vi "Import DPIDs.vi"(8 "error in (no error)":errorcluster, 11 "Node Ptr":u64 format="%.0x") -> (0 "error out":errorcluster)   [LabVIEW 2024, in "Diagnostics Addon System Explorer.lvlib"]
uses:
  Diagnostics Addon System Explorer.lvlib
  Addon Shared/Types/DPID.ctl
  Addon Shared/Types/DPID.Rate.ctl
  Addon Shared/Types/Type.ctl
  <vilib>/Utility/error.llb/Trim Whitespace One-Sided.vi
  <vilib>/NI VeriStand/Custom Device API/Custom Device API.lvlib
  <vilib>/NI VeriStand/Custom Device Tools/Custom Device Utility Library/Custom Device Utility Library.lvlib
  Addon Shared/Diagnostics Addon Shared.lvlib
panel:
  in  "Tag":string
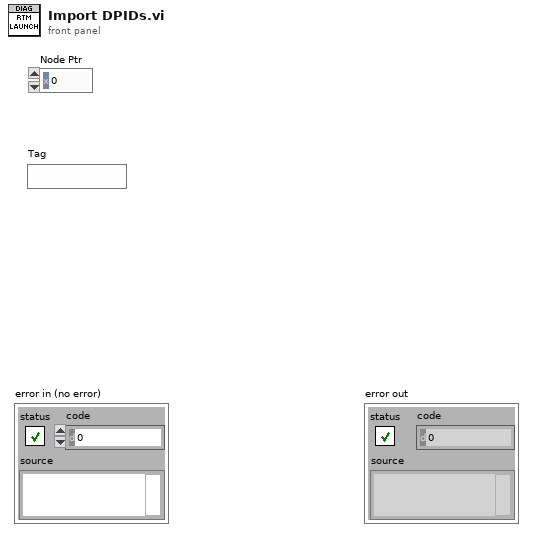
[diagram p1: front panel]
types:
  T1 = typedef "Diagnostics Addon Shared.lvlib/DPID.ctl" = cluster{"DPID ID":u8, "Speed":T2, "PIDs":u16[]}
  T2 = typedef "Diagnostics Addon Shared.lvlib/DPID.Rate.ctl" = enum16{"Slow", "Medium", "Fast"}
  T3 = typedef "Diagnostics Addon Shared.lvlib/Type.ctl" = enum16{"DID", "CDID", "PID", "CPID", "Read Memory", "Write Memory", "IO Control", "Routine Start", "Routine Request", "Routine Stop", "User Defined", "DTC Control", "Clear DTCs", "Read DTCs", "Start DTCs", "DTC Change Count", "Tester Present", "Unlock ECU", "Reset ECU", "Diag Session Control", "Communication Control", "DPID Control", "Poll Control", "Diag Comm Port Control"}
  T4 = typedef "Diagnostics Addon System Explorer.lvlib/Frame.Export.ctl" = cluster{"Name":string, "ID":u32, "Signals":T5[]}
  T5 = typedef "Diagnostics Addon Shared.lvlib/Signal.ctl" = cluster{"Start Bit":u32, "Length":u32, "Scaling Factor":dbl, "Scaling Offset":dbl, "Minimum":dbl, "Maximum":dbl, "Data Type":u32, "Byte Order":u32, "Default Value":dbl, "Name":string, "Units":string}
  T6 = typedef "Custom Device API.lvlib/Custom Device Item Ref.ctl" = u64
  T7 = typedef "Custom Device API.lvlib/Custom Device Item Info.ctl" = cluster{"Name":string, "Is Channel":bool, "GUID":string, "Is Waveform":bool}
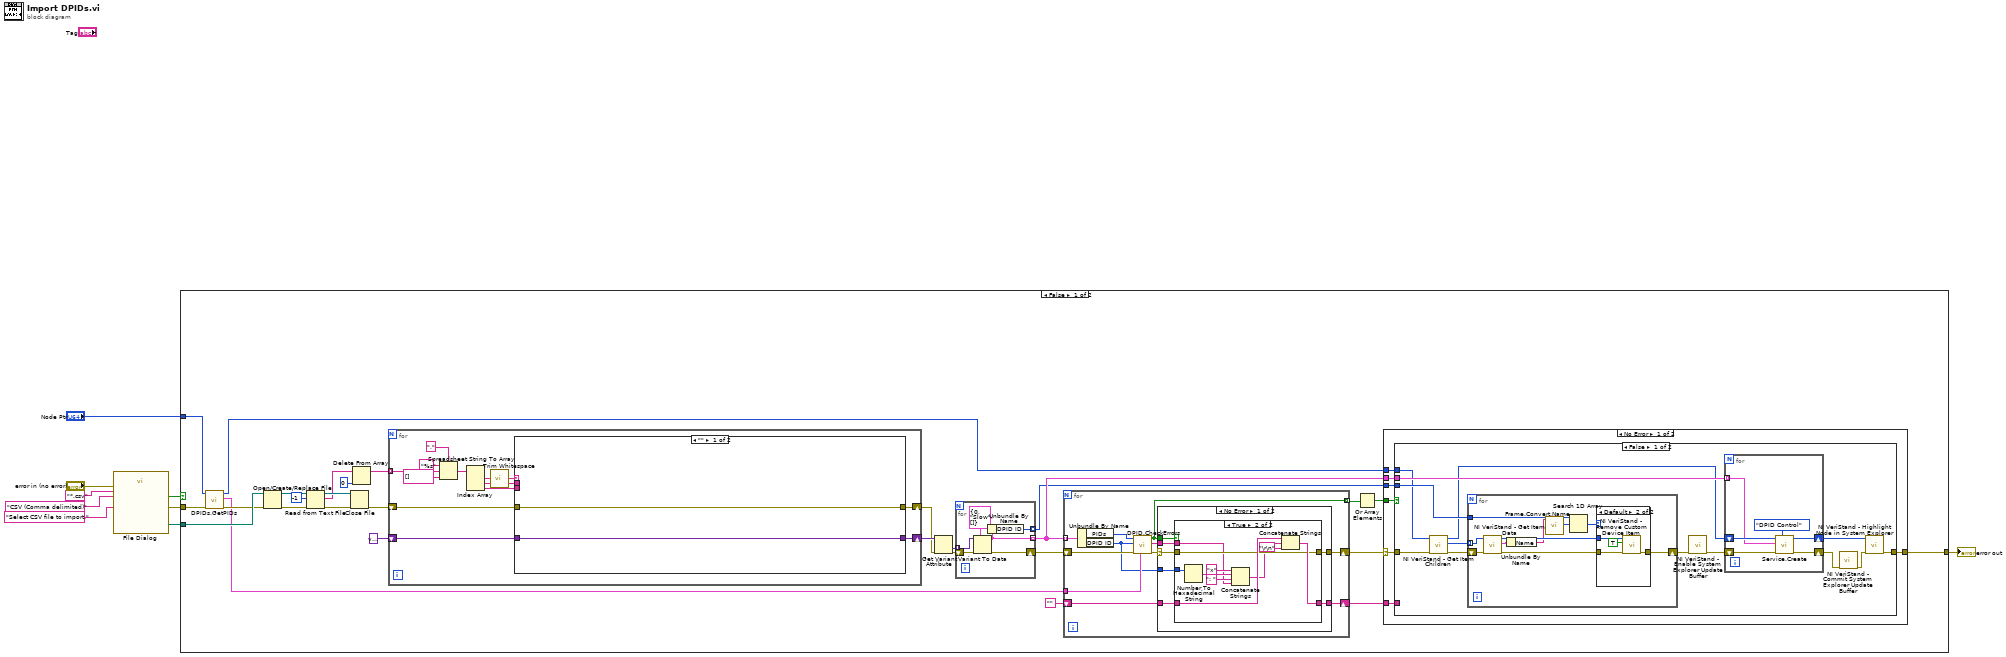
[diagram p0: block diagram]
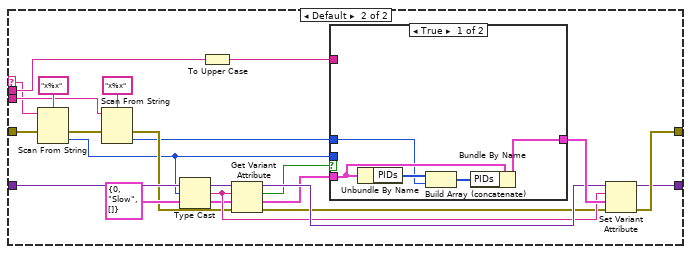
[diagram p2: hidden frame]
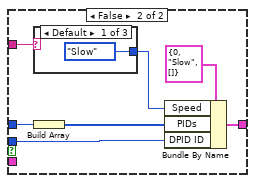
[diagram p3: hidden frame]
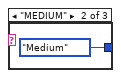
[diagram p4: hidden frame]
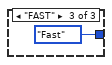
[diagram p5: hidden frame]
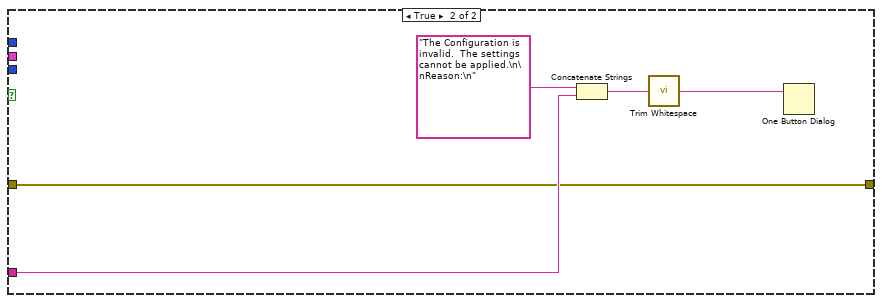
[diagram p7: hidden frame]
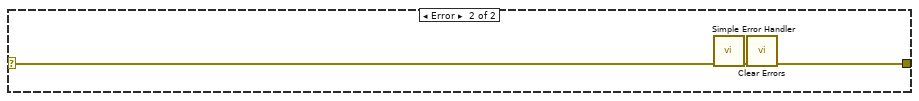
[diagram p8: hidden frame]
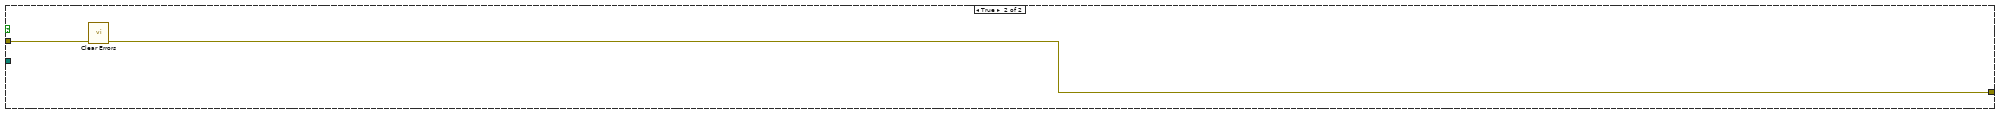
[diagram p11: hidden frame]
diagram:
  n1 = call "File Dialog"("prompt"="Select CSV file to import.", "error in"="error in (no error)", "pattern (all files)"="*.csv" ("pattern label"), "pattern label"="CSV (Comma delimited)") -> ("selected path"=w4:path, "cancelled"=w6:bool, "error out"=w5:errorcluster)  [unwired: 8 in, 1 out]
  n2 = case shown="False" w6 {
    tunnel: w5 -> [w14 w178]
    tunnel: w4 -> [w34 _]
    tunnel: "Node Ptr" -> [w12 _]
    tunnel: [w18 w177] -> w2
    frame False {
      n3 = call "DPIDs.GetPIDs.vi"("error in (no error)"=w14, "Item Ref in"=w12) -> ("error out"=w13:errorcluster, "PIDs"=w10:T4[], "Section Ref out"=w11:T6)  [unwired: 7 in]
      n4 = Open/Create/Replace File(file path (use dialog)=w34, error in=w13) -> (refnum out=w37:refnum<file>, error out=w38:errorcluster)  [unwired: 4 in, 1 out]
      n5 = Read from Text File(file (use dialog)=w37, count=-1, error in=w38) -> (refnum out=w36:refnum<file>, text=w26:string[], error out=w35:errorcluster)  [unwired: 1 in, 1 out]
      n6 = Close File(refnum=w36, error in=w35) -> (error out=w32:errorcluster)  [unwired: 1 out]
      n7 = Delete From Array(array=w26, index=0) -> (array with subset deleted=w25:string[])  [unwired: 1 in, 1 out]
      n8 = for {
        tunnel: w25 -> [w47] mode=indexing
        shift-right: [w49] -> w29
        shift-left: w32 -> [w50]
        shift-right: [w48] -> w30
        shift-left: variant -> [w51]
        n9 = Spreadsheet String To Array(delimiter (Tab)=",", format string="%s", spreadsheet string=w47, array type (2D Dbl)=string[] []) -> (array=w43:string[])
        n10 = Index Array(array=w43) -> (element #1=w40:string, element #2=w41:string, element #3=w42:string)  [unwired: 3 in]
        n11 = call <vilib>:"Trim Whitespace.vi"("string"=w40) -> ("trimmed string"=w39:string)  [unwired: 1 in]
        n12 = case shown="\"\"" w39 {
          selector: w39 -> [_ w54]
          tunnel: w51 -> [w53 w73]
          tunnel: w50 -> [w52 w72]
          tunnel: [w52 w69] -> w49
          tunnel: [w53 w68] -> w48
          tunnel: w42 -> [_ w58]
          tunnel: w41 -> [_ w57]
          frame "" {
          }
          frame Default {
            n13 = Scan From String(format string="x%x", input string=w54, error in=w72) -> (error out=w60:errorcluster, output 1=w55:u32)  [unwired: 2 in, 2 out]
            n14 = Scan From String(format string="x%x", input string=w58, error in=w60) -> (error out=w59:errorcluster, output 1=w56:u32)  [unwired: 2 in, 2 out]
            n15 = Type Cast(x=w55) -> (*(type *) &x=w67:string)  [unwired: 1 in]
            n16 = To Upper Case(1:w57) -> (0:w62:string)
            n17 = Get Variant Attribute(Variant=w73, name=w67, default value (empty Variant)=T1 {"DPID ID"=0, "Speed"=enum."Slow", "PIDs"=[]} ("DPID"), error in=w59) -> (duplicate Variant=w70:variant, found=w66:bool, value=w65:T1, error out=w63:errorcluster)
            n18 = case shown="True" w66 {
              tunnel: w55 -> [_ w80]
              tunnel: w62 -> [_ w82]
              tunnel: [w76 w86] -> w71
              tunnel: w65 -> [w79 _]
              tunnel: w56 -> [w75 w84]
              frame True {
                n19 = Unbundle By Name(w79) -> ("PIDs"=w78:u16[])
                n20 = Build Array (concatenate)(w78, w75) -> (w77:u32[])
                n21 = Bundle By Name(cluster=w79, "PIDs"=w77) -> (w76:T1)
              }
              frame False {
                n22 = case shown="Default" w82 {
                  tunnel: [DPID.Rate."Slow" ("Speed") DPID.Rate."Medium" ("Speed") DPID.Rate."Fast" ("Speed")] -> w81
                  frame Default {
                  }
                  frame "MEDIUM" {
                  }
                  frame "FAST" {
                  }
                }
                n23 = Build Array(w84) -> (w83:u32[])
                n24 = Bundle By Name(cluster=T1 {"DPID ID"=0, "Speed"=enum."Slow", "PIDs"=[]} ("DPID"), "Speed"=w81, "PIDs"=w83, "DPID ID"=w80) -> (w86:T1)
              }
            }
            n25 = Set Variant Attribute(Variant=w70, name=w67, value=w71, error in=w63) -> (Variant out=w68:variant, error out=w69:errorcluster)  [unwired: 1 out]
          }
        }
      }
      n26 = Get Variant Attribute(Variant=w30, error in=w29) -> (values=w28:variant[], error out=w27:errorcluster)  [unwired: 2 in, 2 out]
      n27 = for {
        tunnel: w28 -> [w95] mode=indexing
        shift-right: [w93] -> w17
        shift-left: w27 -> [w94]
        tunnel: [w92] -> w19 mode=indexing
        tunnel: [w91] -> w16 mode=indexing
        n28 = Variant To Data(error in=w94, type=T1 {"DPID ID"=0, "Speed"=enum."Slow", "PIDs"=[]} ("DPID"), Variant=w95) -> (data=w92:T1, error out=w93:errorcluster)
        n29 = Unbundle By Name(w92) -> ("DPID ID"=w91:u8)
      }
      n30 = for {
        tunnel: w19 -> [w155] mode=indexing
        shift-right: [w152] -> w15
        shift-left: w17 -> [w151]
        shift-right: [w154] -> w20
        shift-left: "" -> [w153]
        tunnel: [w148] -> w22 mode=indexing
        tunnel: w10 -> [w147]
        n31 = Unbundle By Name(w155) -> ("PIDs"=w146:u16[], "DPID ID"=w145:u8)
        n32 = call "DPID.CheckErrors.vi"("Existing PIDs"=w147, "error in (no error)"=w151, "DPID ID"=w145, "PIDs"=w146) -> ("error out"=w150:errorcluster, "Reason"=w149:string, "Error?"=w148:bool)  [unwired: 5 in]
        n33 = case shown="No Error" w150 {
          selector: w150 -> [w158 w175]
          tunnel: w148 -> [w161 _]
          tunnel: w149 -> [w162 _]
          tunnel: [w160 w176] -> w154
          tunnel: w153 -> [w159 w176]
          tunnel: [w157 w175] -> w152
          tunnel: w145 -> [w156 _]
          frame No Error {
            n34 = case shown="True" w161 {
              tunnel: w162 -> [_ w166]
              tunnel: [w164 w174] -> w160
              tunnel: w159 -> [w164 w173]
              tunnel: w158 -> [w163 w171]
              tunnel: [w163 w171] -> w157
              tunnel: w156 -> [_ w168]
              frame False {
              }
              frame True {
                n35 = Number To Hexadecimal String(2:w168) -> (0:w170:string)  [unwired: 1 in]
                n36 = Concatenate Strings("x" ("string"), w170, ": " ("string"), w166) -> (w165:string)
                n37 = Concatenate Strings(w173, w165, "\r\n") -> (w174:string)
              }
            }
          }
          frame Error {
          }
        }
      }
      n38 = Or Array Elements(Boolean array=w22) -> (logical OR=w21:bool)
      n39 = case shown="No Error" w15 {
        selector: w15 -> [w98 w144]
        tunnel: w21 -> [w102 _]
        tunnel: w20 -> [w101 _]
        tunnel: w19 -> [w100 _]
        tunnel: [w99 w142] -> w18
        tunnel: w11 -> [w97 _]
        tunnel: w16 -> [w96 _]
        frame No Error {
          n40 = case shown="False" w102 {
            tunnel: w101 -> [_ w139]
            tunnel: w98 -> [w107 w138]
            tunnel: w100 -> [w112 _]
            tunnel: [w111 w138] -> w99
            tunnel: w97 -> [w106 _]
            tunnel: w96 -> [w108 _]
            frame False {
              n41 = call <vilib>:"NI VeriStand - Get Item Children.vi"("error in (no error)"=w107, "Item Ref in"=w106) -> ("error out"=w110:errorcluster, "Child Refs"=w109:T6[], "Item Ref out"=w103:T6)  [unwired: 6 in, 1 out]
              n42 = for {
                shift-right: [w120] -> w105
                shift-left: w110 -> [w124]
                tunnel: w109 -> [w123] mode=indexing
                tunnel: w108 -> [w122]
                n43 = call <vilib>:"NI VeriStand - Get Item Data.vi"("error in (no error)"=w124, "Item Ref in"=w123) -> ("error out"=w121:errorcluster, "Item Info"=w125:T7, "Item Ref out"=w119:T6)  [unwired: 7 out]
                n44 = Unbundle By Name(w125) -> ("Name"=w117:string)
                n45 = call "Frame.Convert.Name.vi"("VS Frame Name"=w117) -> ("ID"=w116:u16)  [unwired: 9 in, 1 out]
                n46 = Search 1D Array(1D array=w122, element=w116) -> (index of element=w118:i32)  [unwired: 1 in]
                n47 = case shown="Default" w118 {
                  tunnel: w121 -> [w126 w130]
                  tunnel: [w126 w129] -> w120
                  tunnel: w119 -> [_ w128]
                  frame -1 {
                  }
                  frame Default {
                    n48 = call <vilib>:"NI VeriStand - Remove Custom Device Item.vi"("error in (no error)"=w130, "Force Delete (F)"=TRUE, "Item Ref in"=w128) -> ("error out"=w129:errorcluster)  [unwired: 7 in, 1 out]
                  }
                }
              }
              n49 = call <vilib>:"NI VeriStand - Enable System Explorer Update Buffer.vi"("error in (no error)"=w105) -> ("error out"=w104:errorcluster)  [unwired: 10 in]
              n50 = for {
                shift-right: [w135] -> w114
                shift-left: w104 -> [w136]
                shift-right: [w133] -> w115
                shift-left: w103 -> [w134]
                tunnel: w112 -> [w132] mode=indexing
                n51 = call "Service.Create.vi"("Type"=Type."DPID Control", "error in (no error)"=w136, "Variant"=w132, "Section Ptr"=w134) -> ("error out"=w135:errorcluster, "Parent Ref out"=w133:T6)  [unwired: 6 in]
              }
              n52 = call <vilib>:"NI VeriStand - Commit System Explorer Update Buffer.vi"("error in (no error)"=w114) -> ("error out"=w113:errorcluster)  [unwired: 10 in]
              n53 = call <vilib>:"NI VeriStand - Highlight Node in System Explorer.vi"("error in (no error)"=w113, "Item Ref in"=w115) -> ("error out"=w111:errorcluster)  [unwired: 8 in, 1 out]
            }
            frame True {
              n54 = Concatenate Strings("The Configuration is invalid.  The settings cannot be applied.\n\nReason:\n" ("message"), w139) -> (w141:string)
              n55 = call <vilib>:"Trim Whitespace.vi"("string"=w141) -> ("trimmed string"=w137:string)  [unwired: 1 in]
              n56 = One Button Dialog(message=w137) -> ()  [unwired: 1 in, 1 out]
            }
          }
        }
        frame Error {
          n57 = call <vilib>:"Simple Error Handler.vi"("error in (no error)"=w144) -> ("error out"=w143:errorcluster)  [unwired: 4 in, 4 out]
          n58 = call <vilib>:"Clear Errors.vi"("error in (no error)"=w143) -> ("error out"=w142:errorcluster)  [unwired: 5 in, 1 out]
        }
      }
    }
    frame True {
      n59 = call <vilib>:"Clear Errors.vi"("error in (no error)"=w178) -> ("error out"=w177:errorcluster)  [unwired: 5 in, 1 out]
    }
  }
  "error out" <- w2
